vi "Add to Balance.vi"() -> ()   [LabVIEW 2015, in "Money.lvlib"]
uses:
  Money.lvlib
panel:
  out "error out":errorcluster
  in  "error in (no error)":errorcluster
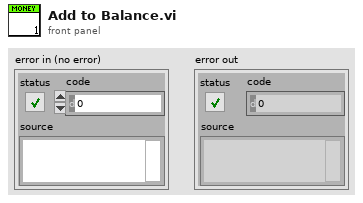
[diagram p1: front panel]
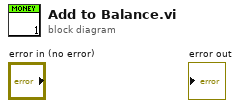
[diagram p0: block diagram]
diagram:
